vi "Get Date Time in Secodns with error cluster.vi"(8 "Error In":errorcluster) -> (0 "Error Out":errorcluster, 2 "current time":timestamp)   [LabVIEW 2017]
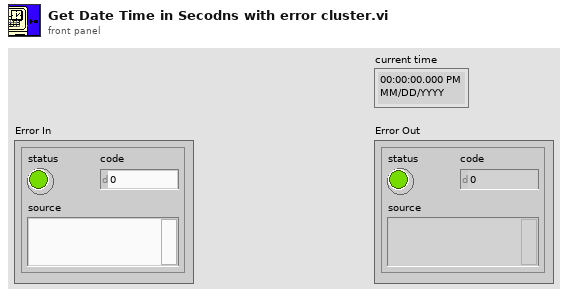
[diagram p1: front panel]
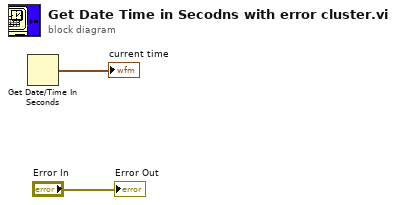
[diagram p0: block diagram]
diagram:
  n1 = Get Date/Time In Seconds() -> (seconds since 1Jan1904=→"current time":timestamp)
  "Error Out" <- "Error In"
